vi "tutorial-rev1.vi"() -> ()   [LabVIEW 2015]
panel:
  in  "error in (no error)":errorcluster
  out "Numeric":dbl
  out "Numeric 2":dbl
  in  "stop":bool
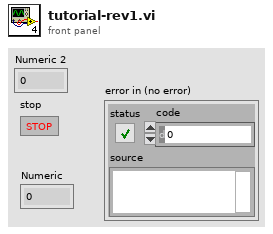
[diagram p1: front panel]
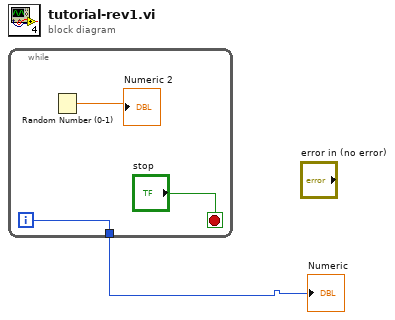
[diagram p0: block diagram]
diagram:
  n1 = while {
    tunnel: [w3] -> w1
    i -> [w3]
    stop <- "stop" stop-if-true
    n2 = Random Number (0-1)() -> (number: 0 to 1=→"Numeric 2":dbl)
  }
  "Numeric" <- w1
